vi "set_maximum_sampling_rate.vi"(8 "error in (no error)":errorcluster, 10 "maximum sampling rate":dbl[unit], 11 "DAQmxWriteSignals.lvclass in":refnum<class "SignalWriterDL090202DAQmx.lvclass">) -> (0 "error out":errorcluster, 3 "DAQmxWriteSignals.lvclass out":refnum<class "SignalWriterDL090202DAQmx.lvclass">)   [LabVIEW 2010, in "SignalWriterDL090202DAQmx.lvclass"]
uses:
  SignalWriterDL090202DAQmx.lvclass
  SignalWriterDL090202DAQmx.lvclass/SignalWriterDL090202DAQmx.ctl
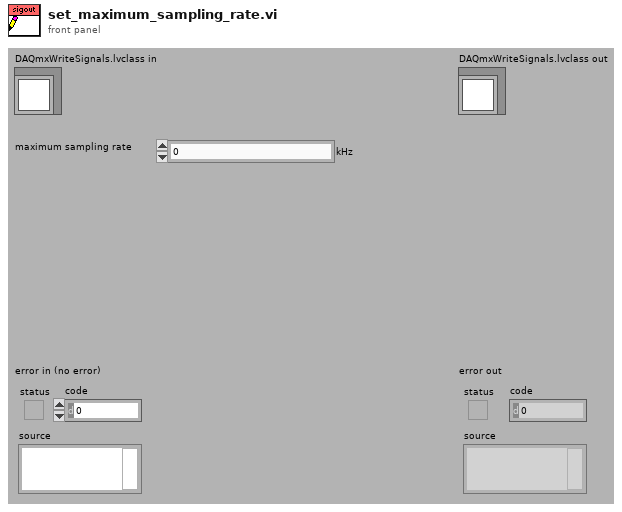
[diagram p1: front panel]
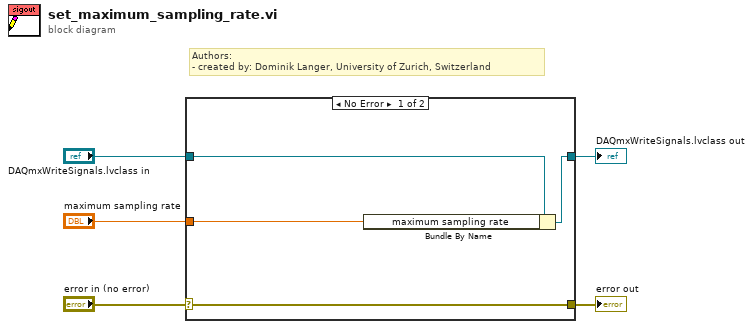
[diagram p0: block diagram]
diagram:
  # "Authors: \n- created by: Dominik Langer, University of Zurich, Switzerland"
  n1 = case shown="No Error" "error in (no error)" {
    selector: "error in (no error)" -> [w9 w10]
    tunnel: [w9 w10] -> w4
    tunnel: [w7 w11] -> w2
    tunnel: "DAQmxWriteSignals.lvclass in" -> [w8 w11]
    tunnel: "maximum sampling rate" -> [w6 _]
    frame No Error {
      n2 = Bundle By Name(cluster=w8, "maximum sampling rate"=w6) -> (w7:refnum<class "SignalWriterDL090202DAQmx.lvclass">)
    }
    frame Error {
    }
  }
  "error out" <- w4
  "DAQmxWriteSignals.lvclass out" <- w2
